vi "instrument.vi"(9 "Amount of Instruments":i32=5, 11 "project-param in":T1) -> (3 "project-param out 3":T1)   [LabVIEW 2019]
uses:
  Project Parameters.ctl
  <vilib>/numeric/Random Number (Range) I64.vi
  <vilib>/numeric/sub_Random U32.vi
panel:
  out "array":string[](array[string])
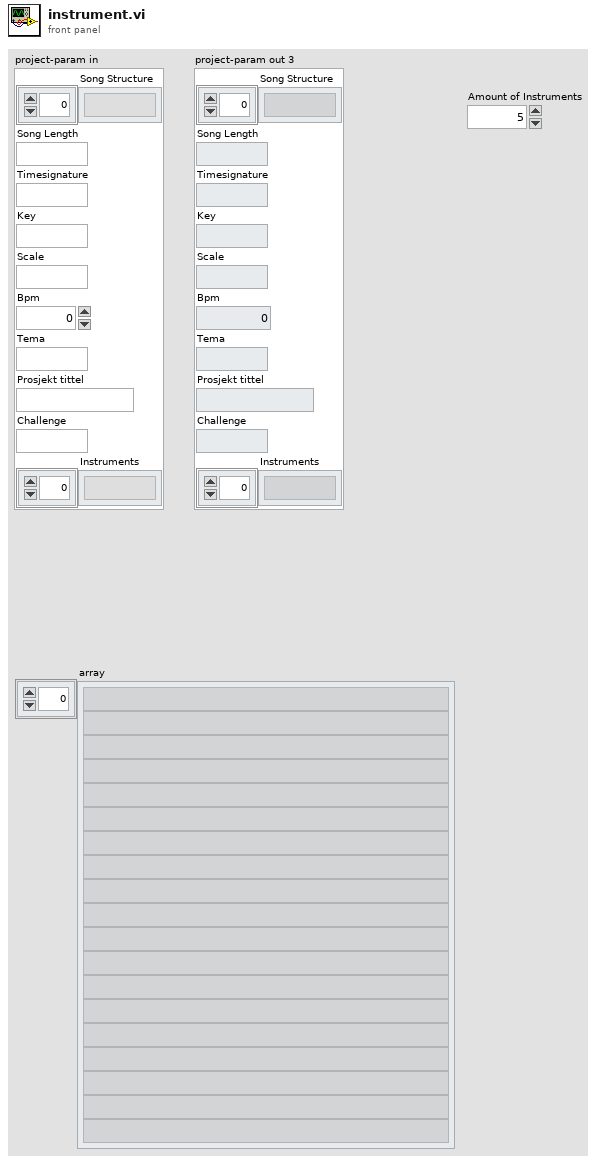
[diagram p1: front panel]
types:
  T1 = typedef "Project Parameters.ctl" = cluster{"Song Structure":string[], "Song Length":string, "Timesignature":string, "Key":string, "Scale":string, "Bpm":i32, "Tema":string, "Prosjekt tittel":string, "Challenge":string, "Instruments":string[]}
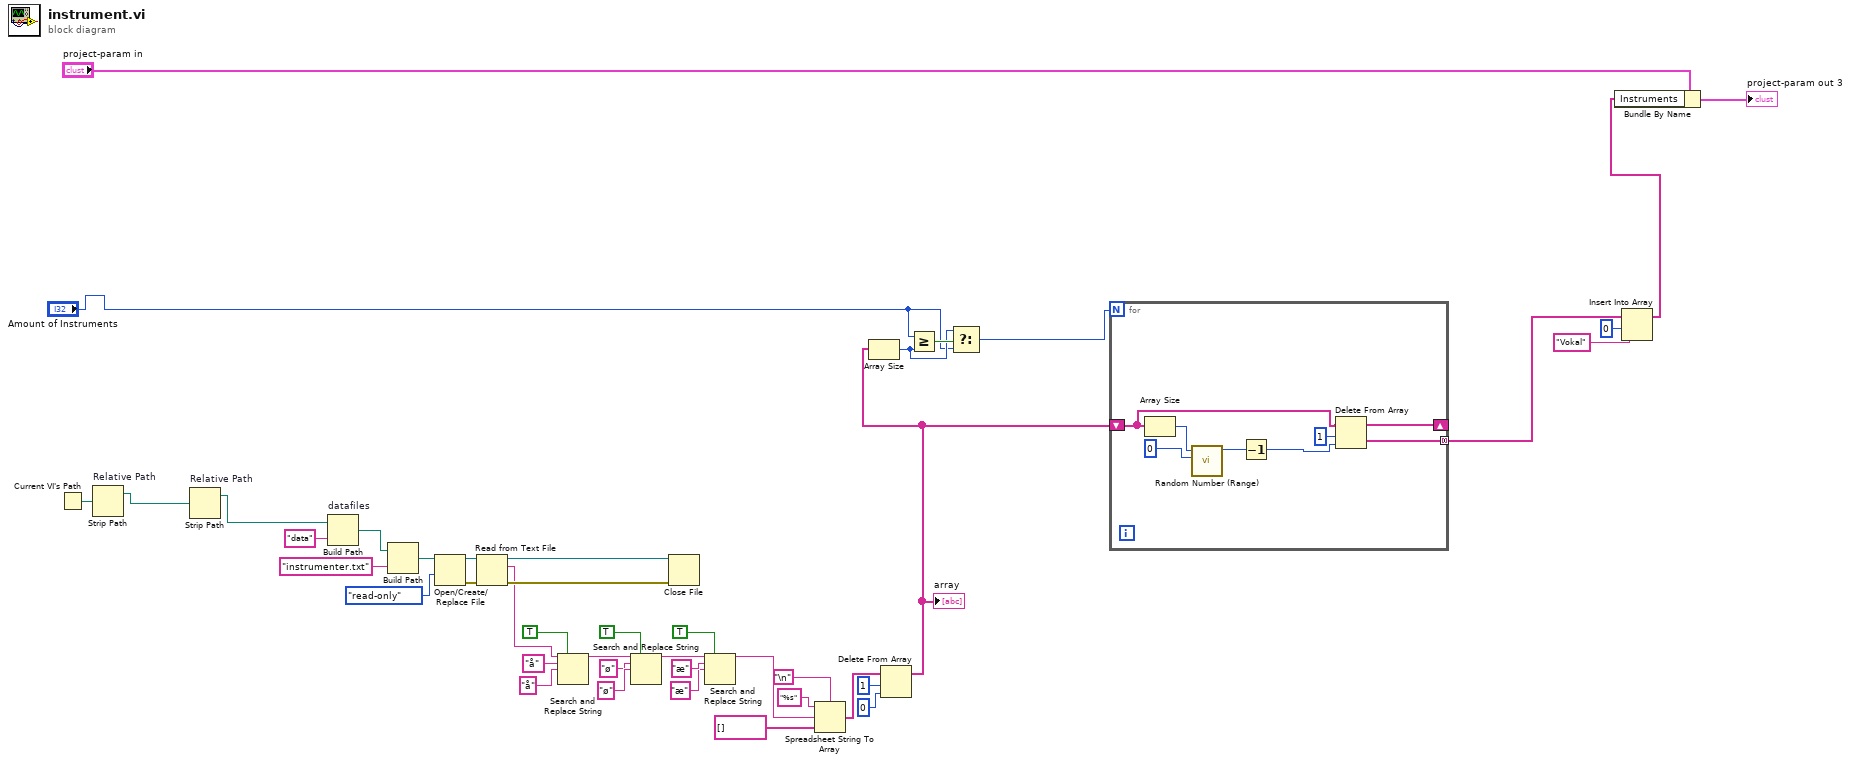
[diagram p0: block diagram]
diagram:
  n1 = Current VI's Path() -> (path=w41:path)
  n2 = Strip Path "Relative Path"(path=w41) -> (stripped path=w6:path)  [unwired: 1 out]
  n3 = Strip Path "Relative Path"(path=w6) -> (stripped path=w5:path)  [unwired: 1 out]
  n4 = Build Path "datafiles"(base path=w5, name or relative path="data") -> (appended path=w33:path)
  n5 = Build Path(base path=w33, name or relative path="instrumenter.txt") -> (appended path=w32:path)
  n6 = Open/Create/Replace File(file path (use dialog)=w32, access (0:read/write)=enum16{"read/write", "read-only", "write-only"}."read-only") -> (refnum out=w38:refnum<file>, error out=w37:errorcluster)  [unwired: 4 in, 1 out]
  n7 = Read from Text File(file (use dialog)=w38, error in=w37) -> (refnum out=w36:refnum<file>, text=w28:string, error out=w35:errorcluster)  [unwired: 2 in, 1 out]
  n8 = Search and Replace String(replace all?=TRUE ("replace all? (F)"), input string=w28, search string="å", replace string="å" ("replace string (\"\")")) -> (result string=w21:string)  [unwired: 4 in, 3 out]
  n9 = Search and Replace String(replace all?=TRUE ("replace all? (F)"), input string=w21, search string="ø", replace string="ø" ("replace string (\"\")")) -> (result string=w17:string)  [unwired: 4 in, 3 out]
  n10 = Close File(refnum=w36, error in=w35) -> ()  [unwired: 2 out]
  n11 = Search and Replace String(replace all?=TRUE ("replace all? (F)"), input string=w17, search string="æ", replace string="æ" ("replace string (\"\")")) -> (result string=w16:string)  [unwired: 4 in, 3 out]
  n12 = Spreadsheet String To Array(delimiter (Tab)="\n", format string="%s", spreadsheet string=w16, array type (2D Dbl)=string[] []) -> (array=w15:string[])
  n13 = Delete From Array(array=w15, length=1, index=0) -> (array with subset deleted=w11:string[])  [unwired: 1 out]
  "array" <- w11
  n14 = Array Size(array=w11) -> (size(s)=w9:i32)
  n15 = Greater Or Equal?(x="Amount of Instruments", y=w9) -> (x >= y?=w10:bool)
  n16 = Select(t=w9, s=w10, f="Amount of Instruments") -> (s? t:f=w7:i32)
  n17 = for {
    N: w7 -> [_]
    shift-right: [w45] -> _
    shift-left: w11 -> [w48]
    tunnel: [w44] -> w4 mode=concatenating
    n18 = Array Size(array=w48) -> (size(s)=w50:i32)
    n19 = call-poly <vilib>:"Random Number (Range).vi"("lower bound (-100)"=i64 0, "upper bound (100)"=w50) -> ("number"=w46:i64)  [unwired: 9 in]
    n20 = Decrement(x=w46) -> (x-1=w43:i64)
    n21 = Delete From Array "Delete From Array"(array=w48, length=1, index=w43) -> (deleted portion=w44:string[], array with subset deleted=w45:string[])
  }
  n22 = Insert Into Array(array=w4, index=0, new element="Vokal" ("new element/subarray")) -> (w1:string[])
  n23 = Bundle By Name(cluster="project-param in", "Instruments"=w1) -> (→"project-param out 3":T1)
